vi "controlContinuousFwd.vi"(7 "Set":bool, 8 "error in":errorcluster, 9 "continous FWD in":bool=TRUE, 10 "axis in":u8, 11 "connection ID":refnum<k5>) -> (0 "error out":errorcluster, 1 "continous FWD out":bool=TRUE, 2 "axis out":u8, 3 "connection ID":refnum<k5>)   [LabVIEW 2016]
doc: "Retrieves the current continuous forward moving status (boolean 'get') or starts/stops continuous forward movement (boolean 'set')"
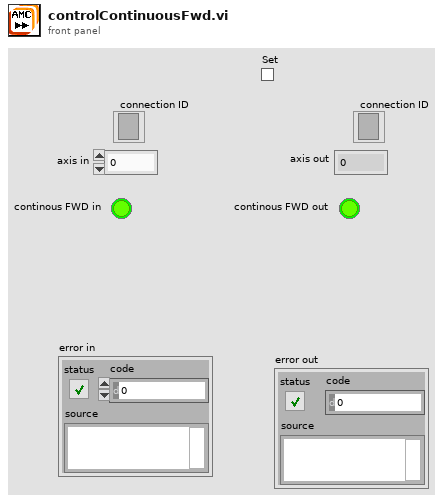
[diagram p1: front panel]
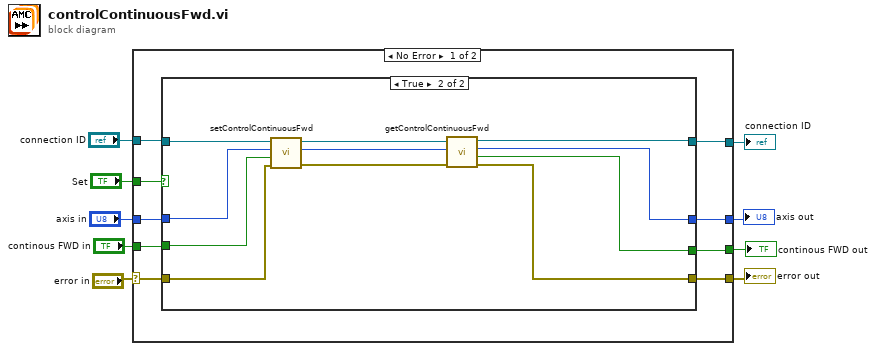
[diagram p0: block diagram]
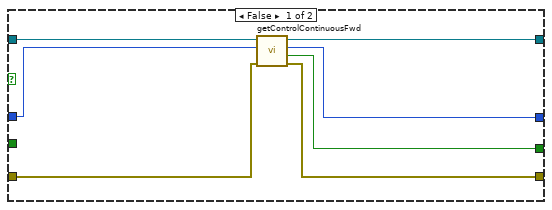
[diagram p2: hidden frame]
diagram:
  n1 = case shown="No Error" "error in" {
    selector: "error in" -> [w10 w40]
    tunnel: "axis in" -> [w15 w38]
    tunnel: [w11 w40] -> w8
    tunnel: [w13 w38] -> w7
    tunnel: "Set" -> [w17 _]
    tunnel: [w12 w39] -> w5
    tunnel: "continous FWD in" -> [w16 w39]
    tunnel: [w14 w37] -> w3
    tunnel: "connection ID" -> [w18 w37]
    frame No Error {
      n2 = case shown="True" w17 {
        tunnel: [w24 w32] -> w14
        tunnel: w18 -> [w25 w36]
        tunnel: w15 -> [w21 w34]
        tunnel: [w19 w31] -> w13
        tunnel: [w22 w30] -> w12
        tunnel: [w23 w29] -> w11
        tunnel: w16 -> [_ w35]
        tunnel: w10 -> [w20 w26]
        frame False {
          n3 = call "getControlContinuousFwd.vi"("error in"=w20, "axis"=w21, "connection ID"=w25) -> ("error out"=w23:errorcluster, "enabled"=w22:bool, "axis_out"=w19:i32, "connection ID"=w24:refnum<k5>)  [unwired: 5 in]
        }
        frame True {
          n4 = call "setControlContinuousFwd.vi"("error in"=w26, "enable"=w35, "axis"=w34, "connection ID"=w36) -> ("error out"=w28:errorcluster, "axis_out"=w27:i32, "connection ID"=w33:refnum<k5>)  [unwired: 5 in]
          n5 = call "getControlContinuousFwd.vi"("error in"=w28, "axis"=w27, "connection ID"=w33) -> ("error out"=w29:errorcluster, "enabled"=w30:bool, "axis_out"=w31:i32, "connection ID"=w32:refnum<k5>)  [unwired: 5 in]
        }
      }
    }
    frame Error {
    }
  }
  "error out" <- w8
  "axis out" <- w7
  "continous FWD out" <- w5
  "connection ID" <- w3
